vi "SequenceState.vi"(7 "LVWSR":refnum<class "Web Request.lvclass">, 11 "st":string) -> ()   [LabVIEW 2017]
uses:
  <vilib>/wsapi/Web Request.lvclass
  Controller/Sequencer/sequenceState.ctl
  Controller/Messages/Change Sequence State MSG/Change Sequence State MSG.lvclass
  C:/Program Files (x86)/National Instruments/LabVIEW 2017/vi.lib/ActorFramework/Message/Message.lvclass
  Controller/Messages/Change Sequence State MSG/Change Sequence State MSG.lvclass/Change Sequence State MSG.ctl
  <vilib>/ActorFramework/Message Enqueuer/Message Enqueuer.lvclass/Message Enqueuer.ctl
  Controller/Messages/Change Sequence State MSG/Write sequence state.vi
  <vilib>/ActorFramework/Message Priority Queue/Priority Enqueue.vi
  Controller/gController.lvclass
  <vilib>/ActorFramework/Message Enqueuer/Message Enqueuer.lvclass
  Controller/Controller.lvlib
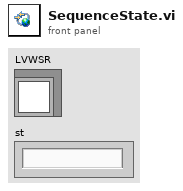
[diagram p1: front panel]
types:
  T1 = typedef "Controller.lvlib/sequenceState.ctl" = enum16{"Run", "Pause", "Reset", "Reload", "Stop"}
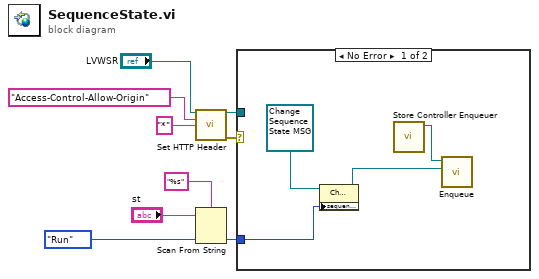
[diagram p0: block diagram]
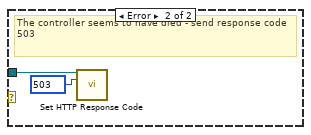
[diagram p2: hidden frame]
diagram:
  n1 = call <vilib>:"Set HTTP Header.vi"("LabVIEW Web Service Request"="LVWSR", "header"="Access-Control-Allow-Origin", "header value"="*") -> ("LabVIEW Web Service Request out"=w7:refnum<class "Web Request.lvclass">, "error out"=w6:errorcluster)  [unwired: 11 in]
  n2 = Scan From String(format string="%s", input string="st", default 1=sequenceState."Run" ("sequence state")) -> (output 1=w1:T1)  [unwired: 2 in, 3 out]
  n3 = case shown="No Error" w6 {
    tunnel: w7 -> [_ w14]
    tunnel: w1 -> [w10 _]
    frame No Error {
      n4 = property class="Change Sequence State MSG"(reference=refnum<class "Change Sequence State MSG.lvclass"> refnum ("Controller.lvlib:Change Sequence State MSG"), "sequence state"=w10) -> (reference out=w11:refnum<class "Change Sequence State MSG.lvclass">)  [unwired: 1 in, 1 out]
      n5 = call "Store Controller Enqueuer.vi"() -> ("Controller Enqueuer Out"=w13:refnum<class "Message Enqueuer.lvclass">)  [unwired: 11 in]
      n6 = call <vilib>:"Enqueue.vi"("Message"=w11, "Message Enqueuer in"=w13) -> ()  [unwired: 8 in, 2 out]
    }
    frame Error {
      w15 = 503 items=["100"=100, "101"=101, "200"=200, "201"=201, "202"=202, "203"=203, "204"=204, "205"=205, "206"=206, "300"=300, "301"=301, "302"=302, "303"=303, "304"=304, "305"=305, "306"=306, "307"=307, "400"=400, "401"=401, "402"=402, "403"=403, "404"=404, "405"=405, "406"=406, "407"=407, "408"=408, "409"=409, "410"=410, "411"=411, "412"=412, "413"=413, "414"=414, "415"=415, "416"=416, "417"=417, "500"=500, "501"=501, "502"=502, "503"=503, "504"=504, "505"=505] ("response code (200)")
      # "The controller seems to have died - send response code 503"
      n7 = call <vilib>:"Set HTTP Response Code.vi"("LabVIEW Web Service Request"=w14, "response code (200)"=w15) -> ()  [unwired: 12 in, 2 out]
    }
  }
